vi "AsyncEngine.CANProtectionAndCounter.vi"(10 "Parameters":variant, 11 "Process":refnum<class "Process.lvclass">) -> ()   [LabVIEW 2019, in "Ghost Bus Addon Engine.lvlib"]
uses:
  Ghost Bus Addon Engine.lvlib
  <vilib>/NI/NIVS Inline Async API/_VS Inline Async API/Process/Process.lvclass
  Types/RT Async Engine Settings.ctl
  Addon Shared/Types/XNET Settings.ctl
  SubModules/Frame-Protection-Support/Source/Engine/Types/RT Frame Settings.ctl
  SubModules/Frame-Protection-Support/Source/Shared/Types/Exported Frame Type.ctl
  SubModules/Frame-Protection-Support/Source/Engine/Types/RT Protection Configuration.ctl
  SubModules/Frame-Protection-Support/Source/Shared/Types/Protection Type.ctl
  SubModules/Frame-Protection-Support/Source/Shared/Types/XNET Signal Configuration.ctl
  SubModules/Frame-Protection-Support/Source/Shared/Types/Exported Counter Settings.ctl
  SubModules/Frame-Protection-Support/Source/Shared/Types/Exported Event Trigger Type.ctl
  SubModules/Frame-Protection-Support/Source/Engine/Types/RT Frame Incoming Values.ctl
  <vilib>/Platform/TimedLoop/XDataNode/timing_clust.ctl
  <vilib>/Platform/TimedLoop/XDataNode/nitl_modes.ctl
  <vilib>/Platform/TimedLoop/XDataNode/wakeup.ctl
  <vilib>/NI/NIVS Inline Async API/_VS Inline Async API/Process/Process.lvclass/Process.ctl
  <vilib>/NI/NIVS Inline Async API/_Data Access Engine/Access Type Classes/Read/Read.lvclass/Read.ctl
  <vilib>/NI/NIVS Inline Async API/_Data Access Engine/Access Type Classes/Write/Write.lvclass/Write.ctl
  <vilib>/NI/NIVS Inline Async API/_VS Inline Async API/Error Handling Process/SubVIs/Error.ConvertArray.vi
  <vilib>/NI/NIVS Inline Async API/_Data Access Engine/Data Access Engine/Methods/Data.Processes.Execute.vi
  <vilib>/NI/NIVS Inline Async API/_Data Access Engine/Data Access Engine/Methods/Write.Data.vi
  SubModules/Frame-Protection-Support/Source/Engine/SubVIs/Calculate Counter And Protections Main Outgoing.vi
  SubModules/Frame-Protection-Support/Source/Engine/SubVIs/Calculate Counter And Protections Main Incoming.vi
  <vilib>/Utility/error.llb/Clear Errors.vi
  SubModules/CAN-Streaming-Support/Source/Addon/Addon Engine/SubVIs/Engine Steam Format Debug String.vi
  SubModules/CAN-Streaming-Support/Source/Addon/Addon Engine/SubVIs/Get Engine Stream Filter.vi
  SubModules/CAN-Streaming-Support/Source/Addon/Addon Engine/SubVIs/CAN Frame Filter.vi
  <vilib>/NI/NIVS Inline Async API/_Data Access Engine/Access Type Classes/Write/Write.ProcessData.vi
  <vilib>/NI/NIVS Inline Async API/_Data Access Engine/Data Access Engine/Methods/Read.Data.Detect.vi
  <vilib>/NI/NIVS Inline Async API/_Data Access Engine/Data Access Engine/Methods/Read.Data.vi
  SubModules/Frame-Protection-Support/Source/Engine/SubVIs/Determine Transmit.vi
  SubModules/Frame-Protection-Support/Source/Engine/SubVIs/Update Counter Signals.vi
  SubModules/Frame-Protection-Support/Source/Engine/SubVIs/Get Frame Data.vi
  SubModules/Frame-Protection-Support/Source/Engine/SubVIs/Convert EU Data to XNET Frame.vi
  SubModules/Frame-Protection-Support/Source/Engine/SubVIs/Update Protection Signals.vi
  SubModules/Frame-Protection-Support/Source/Engine/SubVIs/Determine Disabled.vi
  <vilib>/NI/NIVS Inline Async API/_Data Access Engine/Data Access Engine/Methods/Write.Data.Commit.vi
  SubModules/Frame-Protection-Support/Source/Engine/SubVIs/Get Frame Time Info.vi
  SubModules/Frame-Protection-Support/Source/Engine/SubVIs/Process Regular Signal.vi
  SubModules/Frame-Protection-Support/Source/Engine/SubVIs/Process Counter Signals.vi
  SubModules/Frame-Protection-Support/Source/Engine/SubVIs/Process Protection Signals.vi
  <vilib>/NI/NIVS Inline Async API/_Data Access Engine/Access Type Classes/Write/Write.Buffer.vi
  <vilib>/NI/NIVS Inline Async API/_Data Access Engine/Access Type Classes/Write/Write.Commit.vi
  <vilib>/NI/NIVS Inline Async API/_Data Access Engine/Access Type Classes/Read/Read.ProcessData.Detect.vi
  <vilib>/NI/NIVS Inline Async API/_Data Access Engine/Access Type Classes/Read/Read.ProcessData.vi
  SubModules/Frame-Protection-Support/Source/Engine/SubVIs/Determine Transmission.vi
  SubModules/Frame-Protection-Support/Source/Engine/SubVIs/Determine Periodic.vi
  SubModules/Frame-Protection-Support/Source/Engine/SubVIs/Set Counter Signal.vi
  SubModules/Frame-Protection-Support/Source/Engine/SubVIs/Calculate Counter Value.vi
  SubModules/Frame-Protection-Support/Source/Engine/SubVIs/Set Protection Signal.vi
  SubModules/Frame-Protection-Support/Source/Engine/SubVIs/Calculate Protection Value.vi
  <vilib>/NI/NIVS Inline Async API/_Data Access Engine/Data Access Engine/Methods/Write.Data.Buffer.vi
  SubModules/Frame-Protection-Support/Source/Engine/SubVIs/Get Protection Signals.vi
  <vilib>/xnet/xnet.llb/XNET Create Session.vi
  <vilib>/xnet/xnet.llb/XNET Create Session (Frame Input Stream).vi
  <vilib>/Utility/SystemLogging/Write to System Log.vi
  <vilib>/xnet/xnet.llb/XNET Read.vi
  <vilib>/xnet/xnet.llb/XNET Read (Frame CAN).vi
  <vilib>/xnet/xnet.llb/XNET Read (State CAN Comm).vi
  <vilib>/xnet/xnet.llb/XNET Clear.vi
  <vilib>/xnet/xnet.llb/XNET Convert.vi
  <vilib>/xnet/xnet.llb/XNET Convert (Signal to Frame Raw).vi
  <vilib>/xnet/xnet.llb/XNET Convert (Signal to Frame CAN).vi
  <vilib>/xnet/xnet.llb/XNET Write.vi
  <vilib>/xnet/xnet.llb/XNET Write (Frame CAN).vi
  <vilib>/xnet/xnet.llb/XNET Convert (Frame CAN to Signal).vi
  <vilib>/NI/NI VeriStand Addon Network Comm/Engine/VeriStand Comm.lvclass
  <vilib>/NI/NIVS Inline Async API/_Data Access Engine/Access Type Classes/Write/Write.lvclass
  <vilib>/NI/NIVS Inline Async API/_Data Access Engine/Access Type Classes/Read/Read.lvclass
  <vilib>/Platform/TimedLoop/XDataNode/XDataNode.xnode
  SubModules/Frame-Protection-Support/Source/Shared/Protection and Counter Support Shared.lvlib
  SubModules/Frame-Protection-Support/Source/Engine/Protection and Counter Support Engine.lvlib
  <vilib>/Platform/TimedLoop/XDataNode/XDNodeRunTimeDep.lvlib
  SubModules/CAN-Streaming-Support/Source/Addon/Addon Engine/CAN Stream Support Engine.lvlib
  Addon Shared/Ghost Bus Addon Shared.lvlib
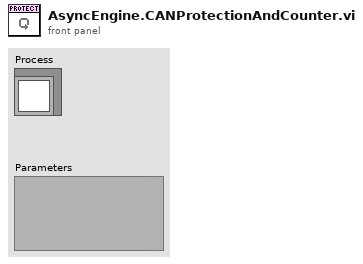
[diagram p1: front panel]
types:
  T1 = typedef "Ghost Bus Addon Engine.lvlib/RT Async Engine Settings.ctl" = cluster{"Name":string, "Priority":i32, "XNET Settings":T2, "FPGA Session":u32, "Outgoing CAN Session":refnum<k21>, "Outgoing Frame Count":i32, "Outgoing Frames":T3[], "Incoming CAN Session":refnum<k21>, "Incoming Frame Count":i32, "Incoming Frames":T3[], "Incoming Values":T10}
  T2 = typedef "Ghost Bus Addon Shared.lvlib/XNET Settings.ctl" = cluster{"Database":refnum<k21>, "Cluster":refnum<k21>, "Port":string, "Baud rate [Bd]":u64, "Termination":u32, "CAN I/O Mode":u32, "FD Baud rate [Bd]":u64, "Priority":i32, "Use Legacy":bool, "FD ISO Mode":u32}
  T3 = typedef "Protection and Counter Support Engine.lvlib/RT Frame Settings.ctl" = cluster{"Type":T4, "Frame ID":u32, "Payload Length":u32, "VS Offset":i32, "VS Length":i32, "Frame Conversion":refnum<k21>, "Frame.Data":dbl[], "Generation Period":u32, "Time Since Last Generation":u32, "Generation Iterations":u32, "Generation Counter":u32, "Has Protection?":bool, "Protection Configurations":T5[], "Has Counter?":bool, "Counter Configurations":T8[], "Has Disable?":bool, "Disable VS Index":i32, "Transmit Trigger":T9, "Trigger VS Index":i32}
  T4 = typedef "Protection and Counter Support Shared.lvlib/Exported Frame Type.ctl" = enum16{"Periodic", "Event", "Periodic/Event"}
  T5 = typedef "Protection and Counter Support Engine.lvlib/RT Protection Configuration.ctl" = cluster{"Protection Frame Index":i32, "Protection Type":T6, "Data Indeces":i32[], "Data Array":dbl[], "Check Sum Conversion":refnum<k21>, "CRC Channels":T7[], "Protection VS Index":i32, "Counter Data Index":i32, "Override Index":i32, "Override Value Index":i32}
  T6 = typedef "Protection and Counter Support Shared.lvlib/Protection Type.ctl" = enum16{"Arb ID + Bytes Checksum with Inversion", "Arb ID + Bytes CRC with Inversion", "Reversed Raw Signal Checksum with Inversion", "Concatenated Two's Compliment"}
  T7 = typedef "Protection and Counter Support Shared.lvlib/XNET Signal Configuration.ctl" = cluster{"Start Bit":i32, "Name":string, "Number of bits":i32, "Scale":dbl, "Offset":dbl, "Data Type":u32, "Counter":bool}
  T8 = typedef "Protection and Counter Support Shared.lvlib/Exported Counter Settings.ctl" = cluster{"Frame Index":i32, "Max Count":dbl, "VS Index":i32, "Bit Length":i64, "Override Index":i32, "Override Value Index":i32}
  T9 = typedef "Protection and Counter Support Shared.lvlib/Exported Event Trigger Type.ctl" = enum16{"Channel value change", "Trigger channel (not zero)", "Channel value change or trigger channel (not zero)", "Trigger channel (any value change)", "Channel value change or trigger channel (any value change)"}
  T10 = typedef "Protection and Counter Support Engine.lvlib/RT Frame Incoming Values.ctl" = cluster{"Signal Values":dbl[], "Signal Invalid Values":dbl[], "ProtCtr Sig Values":dbl[], "Timestamps":timestamp[], "Time Differences":dbl[], "IDs":u32[]}
  T11 = typedef "Ghost Bus Addon Engine.lvlib/RT Async Engine Variables.ctl" = cluster{"Process Ref":refnum<class "Process.lvclass">, "Comm Ref":refnum<class "VeriStand Comm.lvclass">, "Data Refs":T12, "Settings":T1, "Stream Refs":T15}
  T12 = typedef "Ghost Bus Addon Engine.lvlib/RT Data References.ctl" = cluster{"ProtectionsAndCounters.Ref":T13, "Signals.Ref":T14, "Status.Ref":T13, "Overrides":T14, "IncomingSignals.Ref":T13, "CtrandProtctnVld.Ref":T13, "RcvTime.Ref":T13, "TimeDiff.Ref":T13, "IncomingProtCtr.Ref":T13}
  T13 = typedef "Data Access Engine.lvlib/Data Access Engine.lvclass/Write.DVR.ctl" = refnum<data-value>
  T14 = typedef "Data Access Engine.lvlib/Data Access Engine.lvclass/Read.DVR.ctl" = refnum<data-value>
  T15 = typedef "CAN Stream Support Engine.lvlib/Engine Stream Refs.ctl" = cluster{"Addon":string, "Port":refnum<k21>, "Filter Ref":refnum<data-value>, "Default Filter":T16, "Port Settings":T19}
  T16 = typedef "CAN Stream Support Shared.lvlib/Filter Parameters.ctl" = cluster{"ID Filters":u32[], "Direction Filter":T17, "Type Filter":T18}
  T17 = typedef "CAN Stream Support Shared.lvlib/Direction Filter.ctl" = enum16{"Tx/Rx", "Rx", "Tx"}
  T18 = typedef "CAN Stream Support Shared.lvlib/Type Filter.ctl" = enum16{"All", "CAN Data", "CAN Remote", "CAN Bus Error", "CAN 2.0 Data", "CAN FD Data", "CAN FD+BRS Data", "J1939 Data", "Delay", "Log Trigger", "Start Trigger"}
  T19 = typedef "CAN Stream Support Engine.lvlib/Engine Stream Port Settings.ctl" = cluster{"Mode":u32, "Baud Rate":u64, "Termination":u32, "FD ISO Mode":u32, "FD Baud Rate":u64}
  T20 = typedef "XDNodeRunTimeDep.lvlib/timing_clust.ctl" = cluster{"Expected End [f-1]":u64, "Actual End [f-1]":u64, "Finished Late? [f-1]":bool, "Expected End [i-1]":u64, "Actual End [i-1]":u64, "Finished Late? [i-1]":bool, "Expected Start [i]":u64, "Actual Start [i]":u64, "Expected Start [f]":u64, "Actual Start [f]":u64, "Source Name":string, "Structure Name":string, "Period":i64, "Deadline":i64, "Offset":i64, "Start":i64, "Priority":i32, "Timeout":i32, "Mode":T21, "Wakeup Reason":T22, "Error":errorcluster, "Source Type":string, "Secondary Source Type":string, "Global End Time":u64, "Global Start Time":u64, "Frame Duration":u64, "Iteration Duration":u64, "Assigned CPU":i32, "I/O Scan Engine Mode":u32}
  T21 = typedef "XDNodeRunTimeDep.lvlib/nitl_modes.ctl" = enum32{"No Change", "Process missed periods, maintain original phase", "Discard missed periods, maintain original phase", "Process missed periods, ignore original phase", "Discard missed periods, ignore original phase"}
  T22 = typedef "XDNodeRunTimeDep.lvlib/wakeup.ctl" = enum32{"Normal", "Aborted", "Asynchronous wakeup", "Timing source error", "Timed loop error", "Timeout"}
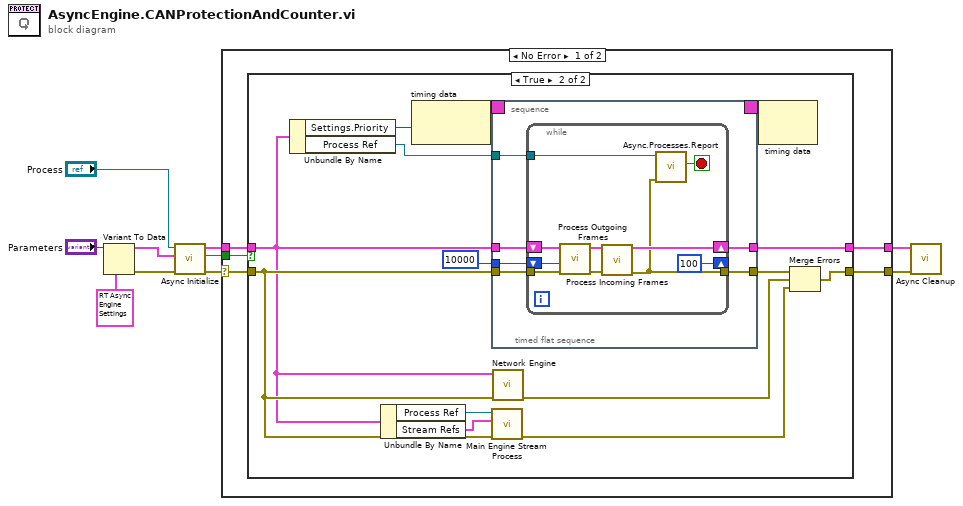
[diagram p0: block diagram]
diagram:
  n1 = Variant To Data(type=T1 {"Name"="", "Priority"=100, "XNET Settings"={"Database"="", "Cluster"="", "Port"="", "Baud rate [Bd]"=0, "Termination"=0, "CAN I/O Mode"=0, "FD Baud rate [Bd]"=500000, "Priority"=100, "Use Legacy"=FALSE, "FD ISO Mode"=0}, "FPGA Session"=0, "Outgoing CAN Session"="", "Outgoing Frame Count"=0, "Outgoing Frames"=[], "Incoming CAN Session"="", "Incoming Frame Count"=0, "Incoming Frames"=[], "Incoming Values"={"Signal Values"=[], "Signal Invalid Values"=[], "ProtCtr Sig Values"=[], "Timestamps"=[], "Time Differences"=[], "IDs"=[]}} ("RT Configuration"), Variant="Parameters") -> (data=w1:T1, error out=w5:errorcluster)  [unwired: 1 in]
  n2 = call "Async Initialize.vi"("error in (no error)"=w5, "RT Configuration"=w1, "Process in"="Process") -> ("error out"=w2:errorcluster, "Execute"=w4:bool, "Variables"=w3:T11)  [unwired: 6 in]
  n3 = case shown="No Error" w2 {
    selector: w2 -> [w14 w61]
    tunnel: w4 -> [w15 _]
    tunnel: [w13 w61] -> w6
    tunnel: [w12 w60] -> w7
    tunnel: w3 -> [w11 w60]
    frame No Error {
      n4 = case shown="True" w15 {
        tunnel: w14 -> [w17 w21]
        tunnel: [w17 w25] -> w13
        tunnel: [w16 w31] -> w12
        tunnel: w11 -> [w16 w19]
        frame False {
        }
        frame True {
          n5 = Unbundle By Name(w19) -> ("Settings.Priority"=w28:i32, "Process Ref"=w27:refnum<class "Process.lvclass">)
          n6 = Unbundle By Name(w19) -> ("Process Ref"=w23:refnum<class "Process.lvclass">, "Stream Refs"=w22:T15)
          n7 = node-c288(w28) -> (w30:T20)
          n8 = timed-sequence {
            timing: w30 -> [_]
            timing-out: [_] -> w29
            tunnel: w27 -> [w33]
            tunnel: w19 -> [w35]
            tunnel: w21 -> [w34]
            tunnel: [w37] -> w18
            tunnel: [w36] -> w31
            tunnel: 10000 ("timeout ms") -> [w32]
            n9 = timed-flat-sequence {
              tunnel: [w39] -> w37
              tunnel: [w40] -> w36
              tunnel: w35 -> [w43]
              tunnel: w34 -> [w42]
              tunnel: w33 -> [w41]
              tunnel: w32 -> [w38]
              n10 = while {
                tunnel: w41 -> [w53]
                tunnel: w42 -> [w52]
                shift-right: [w46] -> w40
                shift-left: w43 -> [w48]
                tunnel: [w44] -> w39
                shift-right: [100 ("timeout ms")] -> _
                shift-left: w38 -> [w50]
                stop <- w51 stop-if-true
                n11 = call "Process Outgoing Frames.vi"("error in (no error)"=w52, "timeout ms"=w50, "Variables"=w48) -> ("error out"=w47:errorcluster, "Variables out"=w45:T11)  [unwired: 7 in]
                n12 = call "Process Incoming Frames.vi"("Variables In"=w45, "error in"=w47) -> ("Variables Out"=w46:T11, "error out"=w44:errorcluster)  [unwired: 12 in]
                n13 = call <vilib>:"Async.Processes.Report.vi"("Error"=w44, "Process in"=w53) -> ("Stop"=w51:bool)  [unwired: 8 in, 1 out]
              }
            }
          }
          n14 = call "Main Engine Stream Process.vi"("error in (no error)"=w21, "Refs"=w22, "Process in"=w23) -> ("error out"=w20:errorcluster)  [unwired: 8 in]
          n15 = call "Network Engine.vi"("error in (no error)"=w21, "Variables"=w19) -> ("error out"=w24:errorcluster)  [unwired: 9 in]
          n16 = node-c288(w29) -> ()  [unwired: 1 out]
          n17 = Merge Errors(w18, w24, w20) -> (w25:errorcluster)
        }
      }
    }
    frame Error {
    }
  }
  n18 = call "Async Cleanup.vi"("error in (no error)"=w6, "Variables"=w7) -> ()  [unwired: 9 in, 1 out]
